vi "RPN to Infix.vi"(11 "Array 2":T1[](array[typedef])) -> (3 "element":string)   [LabVIEW 2018, in "RPN.lvlib"]
uses:
  RPN.lvlib
  Node Type Def.ctl
  <vilib>/Utility/Data Type/NI_Data Type.lvlib
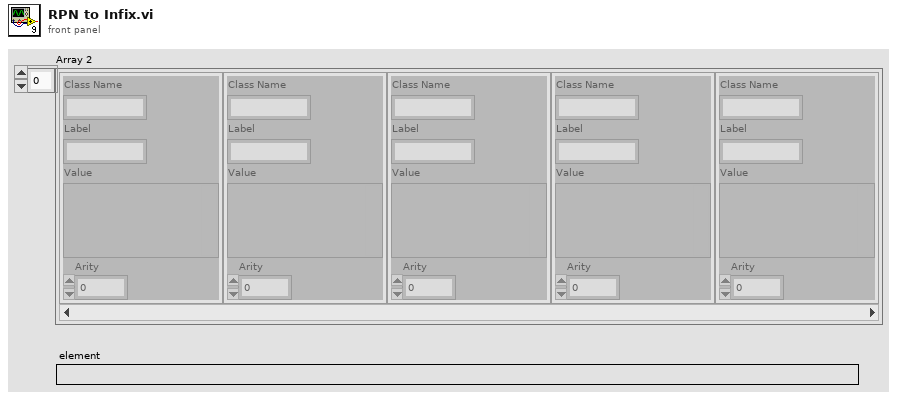
[diagram p1: front panel]
types:
  T1 = typedef "RPN.lvlib/Node Type Def.ctl" = cluster{"Class Name":string, "Label":string, "Value":variant, "Arity":u8}
  T2 = typedef "NI_Data Type.lvlib/Data Type.ctl" = enum8{"Invalid Type", "Void", "I8", "I16", "I32", "I64", "U8", "U16", "U32", "U64", "Single Float", "Double Float", "Extended Float", "Single Complex", "Double Complex", "Extended Complex", "Enum U8", "Enum U16", "Enum U32", "Enum U64", "Single Float With Unit", "Double Float With Unit", "Extended Float With Unit", "Single Complex with Unit", "Double Complex with Unit", "Extended Complex with Unit", "Boolean", "String", "Path", "Picture", "Tag", "Array", "Cluster", "Variant", "LV Variant", "Waveform", "Timestamp", "Digital Waveform", "Digital Data", "ExpressData", "Refnum", "External Data", "VI", "Poly VI", "LabVIEW Class Instance", "Fixed Point"}
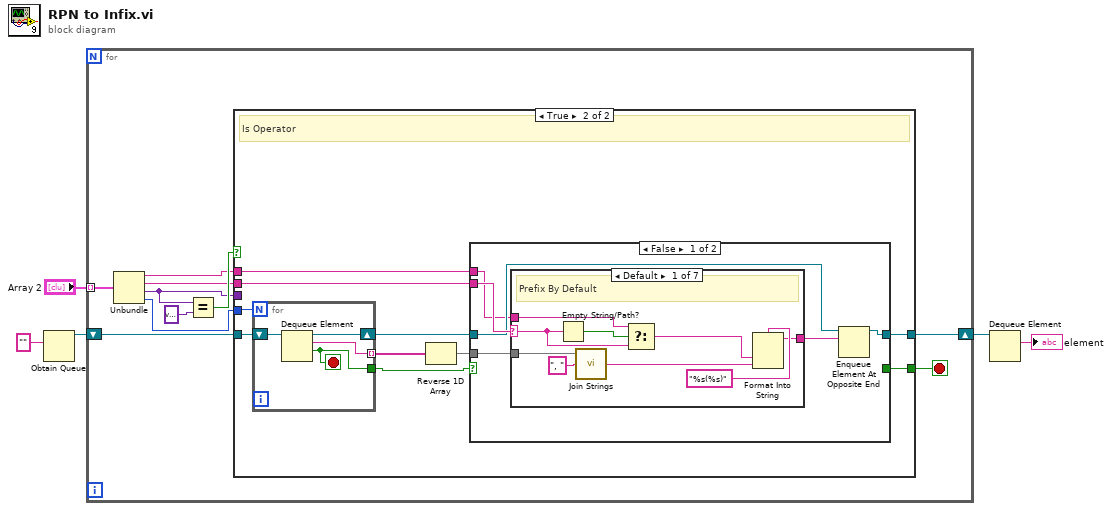
[diagram p0: block diagram]
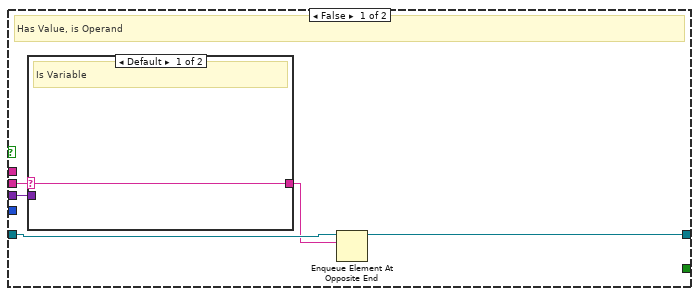
[diagram p2: hidden frame]
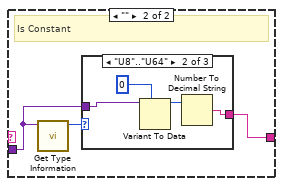
[diagram p3: hidden frame]
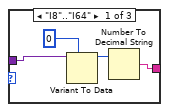
[diagram p4: hidden frame]
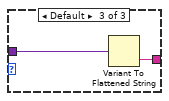
[diagram p5: hidden frame]
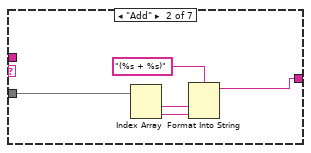
[diagram p6: hidden frame]
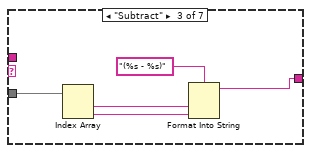
[diagram p7: hidden frame]
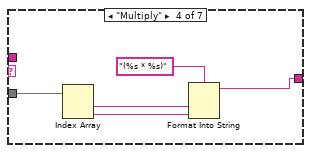
[diagram p8: hidden frame]
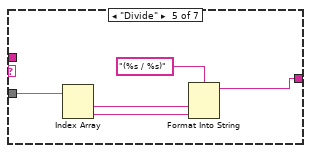
[diagram p9: hidden frame]
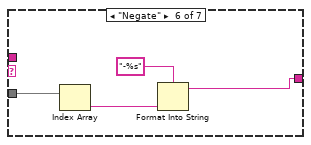
[diagram p10: hidden frame]
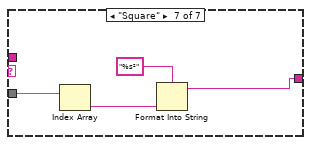
[diagram p11: hidden frame]
diagram:
  n1 = Obtain Queue(element data type="" ("String")) -> (queue out=w4:refnum<queue>)  [unwired: 4 in, 2 out]
  n2 = for {
    tunnel: "Array 2" -> [w15] mode=indexing
    shift-right: [w8] -> w3
    shift-left: w4 -> [w10]
    stop <- w6 stop-if-true
    n3 = Unbundle(w15) -> ("Class Name"=w11:string, "Label"=w12:string, "Value"=w9:variant, "Arity"=w7:u8)
    n4 = Equal?(x=w9, y=variant) -> (x = y?=w13:bool)
    n5 = case shown="True" w13 {
      tunnel: w12 -> [w19 w38]
      tunnel: w11 -> [_ w35]
      tunnel: w10 -> [w17 w43]
      tunnel: w9 -> [w20 _]
      tunnel: [w18 w44] -> w8
      tunnel: w7 -> [_ w41]
      tunnel: [_ w37] -> w6
      frame False {
        # "Has Value, is Operand"
        n6 = case shown="Default" w19 {
          selector: w19 -> [w21 _]
          tunnel: w20 -> [_ w23]
          tunnel: [w21 w22] -> w16
          frame Default {
            # "Is Variable"
          }
          frame "" {
            # "Is Constant"
            n7 = call <vilib>:"Get Type Information.vi"("Variant"=w23) -> ("Type"=w24:T2)  [unwired: 6 in, 4 out]
            n8 = case shown="\"U8\"..\"U64\"" w24 {
              tunnel: w23 -> [w28 w32 w34]
              tunnel: [w25 w29 w33] -> w22
              frame "I8".."I64" {
                n9 = Variant To Data(type=i64 0, Variant=w28) -> (data=w26:i64)  [unwired: 1 in, 1 out]
                n10 = Number To Decimal String(number=w26) -> (decimal integer string=w25:string)  [unwired: 1 in]
              }
              frame "U8".."U64" {
                n11 = Variant To Data(type=u64 0, Variant=w32) -> (data=w30:u64)  [unwired: 1 in, 1 out]
                n12 = Number To Decimal String(number=w30) -> (decimal integer string=w29:string)  [unwired: 1 in]
              }
              frame Default {
                n13 = Variant To Flattened String(Variant=w34) -> (data string=w33:string)  [unwired: 1 out]
              }
            }
          }
        }
        n14 = Enqueue Element At Opposite End(queue=w17, element=w16) -> (queue out=w18:refnum<queue>)  [unwired: 2 in, 2 out]
      }
      frame True {
        # "Is Operator"
        n15 = for {
          N: w41 -> [_]
          shift-right: [w47] -> w42
          shift-left: w43 -> [w48]
          tunnel: [w46] -> w40
          tunnel: [w45] -> w39 mode=indexing
          stop <- w46 stop-if-true
          n16 = Dequeue Element(queue=w48) -> (queue out=w47:refnum<queue>, element=w45:string, timed out?=w46:bool)  [unwired: 2 in, 1 out]
        }
        n17 = Reverse 1D Array(array=w39) -> (reversed array=w36:string[])
        n18 = case shown="False" w40 {
          selector: w40 -> [_ w92]
          tunnel: w42 -> [w52 w93]
          tunnel: [w51 w93] -> w44
          tunnel: w36 -> [w53 _]
          tunnel: w38 -> [w54 _]
          tunnel: [_ w92] -> w37
          tunnel: w35 -> [w49 _]
          frame False {
            n19 = case shown="Default" w54 {
              selector: w54 -> [w56 _ _ _ _ _ _]
              tunnel: w53 -> [w63 w67 w72 w77 w82 w86 w90]
              tunnel: [w59 w64 w69 w74 w79 w84 w88] -> w50
              tunnel: w49 -> [w57 _ _ _ _ _ _]
              frame Default {
                # "Prefix By Default"
                n20 = Empty String/Path?(string/path=w56) -> (empty?=w58:bool)
                n21 = call <vilib>:"Join Strings.vi"("Separator (,)"=", ", "Strings In"=w63) -> ("String"=w61:string)  [unwired: 1 in]
                n22 = Select(t=w57, s=w58, f=w56) -> (s? t:f=w55:string)
                n23 = Format Into String(format string="%s(%s)", w55, w61) -> (resulting string=w59:string)  [unwired: 2 in, 1 out]
              }
              frame "Add" {
                n24 = Index Array(array=w67) -> (element #1=w66:string, element #2=w65:string)  [unwired: 2 in]
                n25 = Format Into String(format string="(%s + %s)", w66, w65) -> (resulting string=w64:string)  [unwired: 2 in, 1 out]
              }
              frame "Subtract" {
                n26 = Index Array(array=w72) -> (element #1=w71:string, element #2=w70:string)  [unwired: 2 in]
                n27 = Format Into String(format string="(%s - %s)", w71, w70) -> (resulting string=w69:string)  [unwired: 2 in, 1 out]
              }
              frame "Multiply" {
                n28 = Index Array(array=w77) -> (element #1=w76:string, element #2=w75:string)  [unwired: 2 in]
                n29 = Format Into String(format string="(%s * %s)", w76, w75) -> (resulting string=w74:string)  [unwired: 2 in, 1 out]
              }
              frame "Divide" {
                n30 = Index Array(array=w82) -> (element #1=w81:string, element #2=w80:string)  [unwired: 2 in]
                n31 = Format Into String(format string="(%s / %s)", w81, w80) -> (resulting string=w79:string)  [unwired: 2 in, 1 out]
              }
              frame "Negate" {
                n32 = Index Array(array=w86) -> (element=w85:string)  [unwired: 1 in]
                n33 = Format Into String(format string="-%s", w85) -> (resulting string=w84:string)  [unwired: 2 in, 1 out]
              }
              frame "Square" {
                n34 = Index Array(array=w90) -> (element=w89:string)  [unwired: 1 in]
                n35 = Format Into String(format string="%s²", w89) -> (resulting string=w88:string)  [unwired: 2 in, 1 out]
              }
            }
            n36 = Enqueue Element At Opposite End(queue=w52, element=w50) -> (queue out=w51:refnum<queue>)  [unwired: 2 in, 2 out]
          }
          frame True {
            # "/* input not sufficient values in the expression */"
          }
        }
      }
    }
  }
  n37 = Dequeue Element(queue=w3) -> (element=→"element":string)  [unwired: 2 in, 3 out]
